vi "Login.vi"(8 "error in (no error)":errorcluster) -> (0 "error out":errorcluster, 2 "Login Successed":bool, 3 "UserName":string)   [LabVIEW 2018]
doc: "Login Form\n\nGet user data from Logins.txt. It is a .iniconfiguration file with Login section where each item has the form:\nUserId=Password,USerName"
uses:
  <vilib>/Utility/config.llb/Read Key (String).vi
  <vilib>/Utility/error.llb/Error Cluster From Error Code.vi
  <vilib>/ErrorRing/Error Ring.xnode
  <vilib>/Utility/config.llb/NI_LVConfig.lvlib
panel:
  out "Color Box":u32(colorbox)
  in  "UserID":string
  in  "Password":string
  in  "stop":bool
  in  "Login":bool
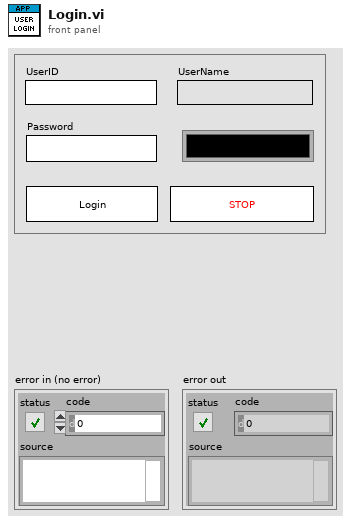
[diagram p1: front panel]
types:
  T1 = enum32{"Invalid", "Standard", "Closed", "Hidden", "Minimized", "Maximized"}
  T2 = typedef "NI_LVConfig.lvlib/Config Data RefNum.ctl" = refnum<k1>
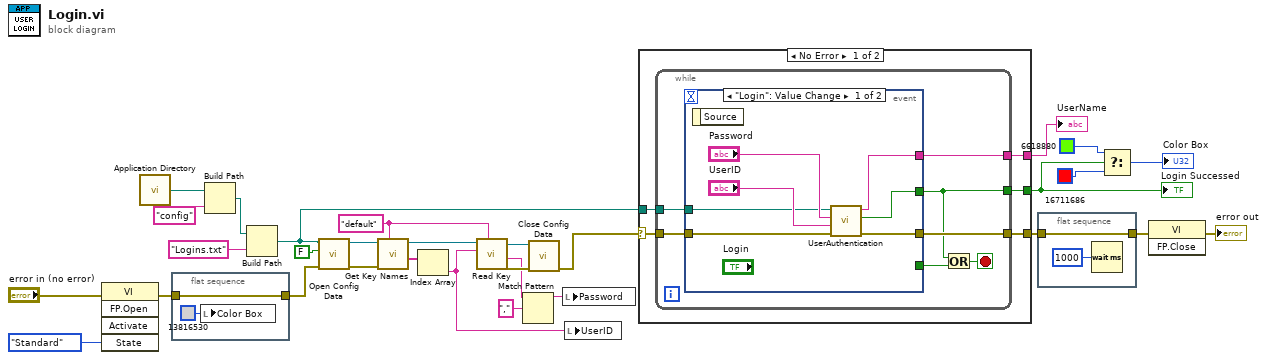
[diagram p0: block diagram]
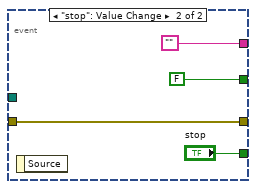
[diagram p2: hidden frame]
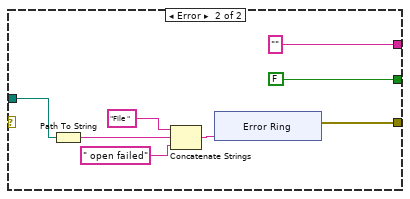
[diagram p3: hidden frame]
diagram:
  w9 = "default" ("section")
  n1 = invoke class="VI" method="FP.Open"(error in="error in (no error)", "State"=T1."Standard") -> (error out=w20:errorcluster)  [unwired: 3 in, 4 out]
  n2 = call <vilib>:"Application Directory.vi"() -> ("Application Directory"=w18:path)
  n3 = flat-sequence {
    tunnel: [w31] -> w13
    tunnel: w20 -> [w31]
    frame #0 {
      n4 = local write "Color Box"(u32 13816530 ("Color Box")) -> ()
    }
  }
  n5 = Build Path(base path=w18, name or relative path="config") -> (appended path=w17:path)
  n6 = Build Path(base path=w17, name or relative path="Logins.txt") -> (appended path=w15:path)
  n7 = call <vilib>:"Open Config Data.vi"("error in (no error)"=w13, "create file if necessary (T)"=FALSE, "configuration file path"=w15) -> ("error out"=w12:errorcluster, "refnum"=w11:T2)  [unwired: 6 in, 1 out]
  n8 = call <vilib>:"Get Key Names.vi"("section"=w9, "error in (no error)"=w12, "refnum"=w11) -> ("key names"=w1:string[], "refnum out"=w10:T2)  [unwired: 5 in, 2 out]
  n9 = Index Array(array=w1) -> (element=w5:string)  [unwired: 1 in]
  n10 = call-poly <vilib>:"Read Key.vi"("section"=w9, "key"=w5, "refnum"=w10) -> ("error out"=w8:errorcluster, "value"=w4:string, "refnum out"=w6:T2)  [unwired: 5 in, 1 out]
  n11 = Match Pattern(string=w4, regular expression=",") -> (before substring=w2:string)  [unwired: 1 in, 3 out]
  n12 = call <vilib>:"Close Config Data.vi"("error in (no error)"=w8, "refnum"=w6) -> ("error out"=w7:errorcluster)  [unwired: 8 in, 1 out]
  n13 = local write "Password"(w2) -> ()
  n14 = local write "UserID"(w5) -> ()
  n15 = case shown="No Error" w7 {
    selector: w7 -> [w33 _]
    tunnel: w15 -> [w37 w62]
    tunnel: [w35 "" ("value")] -> w29
    tunnel: [w34 FALSE ("Visible")] -> w24
    tunnel: [w36 w56] -> w26
    frame No Error {
      n16 = while {
        tunnel: w37 -> [w44]
        tunnel: [w41] -> w36
        tunnel: [w40] -> w35
        tunnel: [w39] -> w34
        tunnel: w33 -> [w38]
        stop <- w42 stop-if-true
        n17 = event shown="[0] \"Login\": Value Change" {
          selector: _ -> [_ _]
          dyn-events: _ -> [_ _]
          timeout: _ -> [_ _]
          tunnel: [w51 w52] -> w41
          tunnel: [_ "stop"] -> w43
          tunnel: w44 -> [w48 _]
          tunnel: [w47 ""] -> w40
          tunnel: w38 -> [w46 w52]
          tunnel: [w45 FALSE ("Boolean")] -> w39
          event "Login": Value Change {
            n18 = event-data() -> ()  [unwired: 1 in, 1 out]
            n19 = call "UserAuthentication.vi"("error in (no error)"=w46, "UserID"="UserID", "Password"="Password", "path"=w48) -> ("error out"=w51:errorcluster, "Boolean"=w45:bool, "UserName"=w47:string)  [unwired: 5 in]
          }
          event "stop": Value Change {
            n20 = event-data() -> ()  [unwired: 1 in, 1 out]
          }
        }
        n21 = Or(x=w39, y=w43) -> (x .or. y?=w42:bool)
      }
    }
    frame Error {
      n22 = Path To String(path=w62) -> (string=w60:string)
      n23 = Concatenate Strings("File " ("string"), w60, " open failed" ("string")) -> (w57:string)
      n24 = xnode "Error Ring"("parameter 0"=w57) -> ("error out"=w56:errorcluster)
    }
  }
  "UserName" <- w29
  "Login Successed" <- w24
  n25 = flat-sequence {
    tunnel: w26 -> [w72]
    tunnel: [w72] -> w25
    frame #0 {
      n26 = Wait (ms)(milliseconds to wait=u32 1000) -> ()  [unwired: 1 out]
    }
  }
  n27 = Select(t=u32 6618880 ("Color Box"), s=w24, f=u32 16711686 ("Color Box")) -> (s? t:f=→"Color Box":u32)
  n28 = invoke class="VI" method="FP.Close"(error in=w25) -> (error out=→"error out":errorcluster)  [unwired: 2 in, 2 out]
